vi "BRig_RT__Case_Exp__recordAnalogInput__PortC__dataQ.vi"(0 "input_dataAnalog":u16[][](array[numeric]), 1 "input_index":i32, 2 "input_iOccurence":u16, 3 "resetOccurrence":bool, 4 "input_dataCurrent":u16[](array[numeric]), 5 "input_stateList_NoInterrupt":u16[](array[numeric]), 6 "input_iState_start":T1, 7 "input_dataQ_hdl":refnum<queue>, 8 "input_iState_end":T1, 9 "input_dataQ_error":errorcluster, 10 "input_AI1":i16, 12 "input_AI0":i16) -> (11 "output_dataQ_error":errorcluster, 13 "output_dataQ_hdl":refnum<queue>, 14 "output_dataAnalog":u16[][](array[numeric]), 15 "output_index":i32, 16 "output_iOccurrence":u16)   [LabVIEW 2014]
uses:
  myRIO_BRig_RT__Case_Exp_stateList.ctl
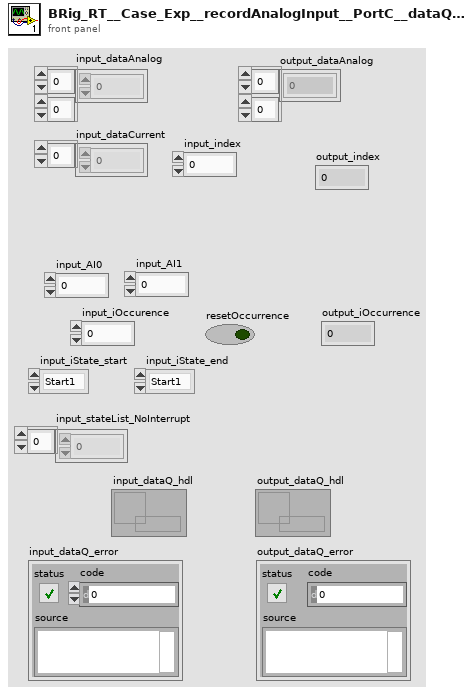
[diagram p1: front panel]
types:
  T1 = typedef "myRIO_BRig_RT__Case_Exp_stateList.ctl" = enum16{"Start1", "Start2", "Start3", "saveSettings1", "saveSettings2", "saveSettings3", "saveSettings4", "saveSettings_LC_ENL_l1", "saveSettings_LC_ENL_l2", "saveSettings_LC_Cue_l1", "saveSettings_LC_Cue_l2", "saveSettings6_LC_l1_Other", "SaveSettings6_LC_l2_Other", "setSettings_Audio", "setSettings_Laser", "initBlock_pre", "initBlock", "initBlock2", "initBlock_post", "initTrial_pre", "initTrial", "initTrial2", "initTrial3", "initTrial4", "initTrial_LC_ENL1", "initTrial_LC_Cue1", "initTrial_LC_Cue1_2", "initTrial_LC_Sel", "initTrial_post", "ENL1_pre", "ENL1", "ENL1_post", "ENL1Penalty_pre", "ENL1Penalty", "ENL2_pre", "ENL2", "ENL2Penalty_pre", "ENL2Penalty", "Cue1_pre", "Cue1", "Cue1_post", "Cue1Penalty_pre", "Cue1Penalty", "Cue2_pre", "Cue2", "Cue2Penalty_pre", "Cue2Penalty", "Selection_pre", "Selection", "Select_post", "SelectReward_pre", "SelectReward", "SelectRewardPost_pre", "SelectRewardPost", "SelectWrong_pre", "SelectWrong", "SelectWrong_post", "SelectTimeout_pre", "SelectTimeout", "SelectTimeout_post", "endTrial_pre", "endTrial1", "endTrial2", "endTrial3", "endTrial_post", "endBlock_pre", "endBlock", "endBlock_post", "endExp", "commConnect", "commUpload_pre", "commUpload_dataBlock", "commUpload_dataCurrent", "commUpload_dataExp", "commUpload_dataLC", "commUpload_dataTrial", "commUpload_post", "saveData_pre", "saveData_dataBlock", "saveData_dataCurrent", "saveData_dataExp", "saveData_dataLC", "saveData_dataTrial", "saveData_post", "empty_endBlock1", "empty_endBlock2", "empty_endTrial1", "empty_endTrial2", "empty_endTrial3", "empty_endTrial4", "empty_endTrial5", "dummyState", "dummyState_endBlock", "FreeReward_pre", "FreeReward", "FreeRewardPost_pre", "FreeRewardPost"}
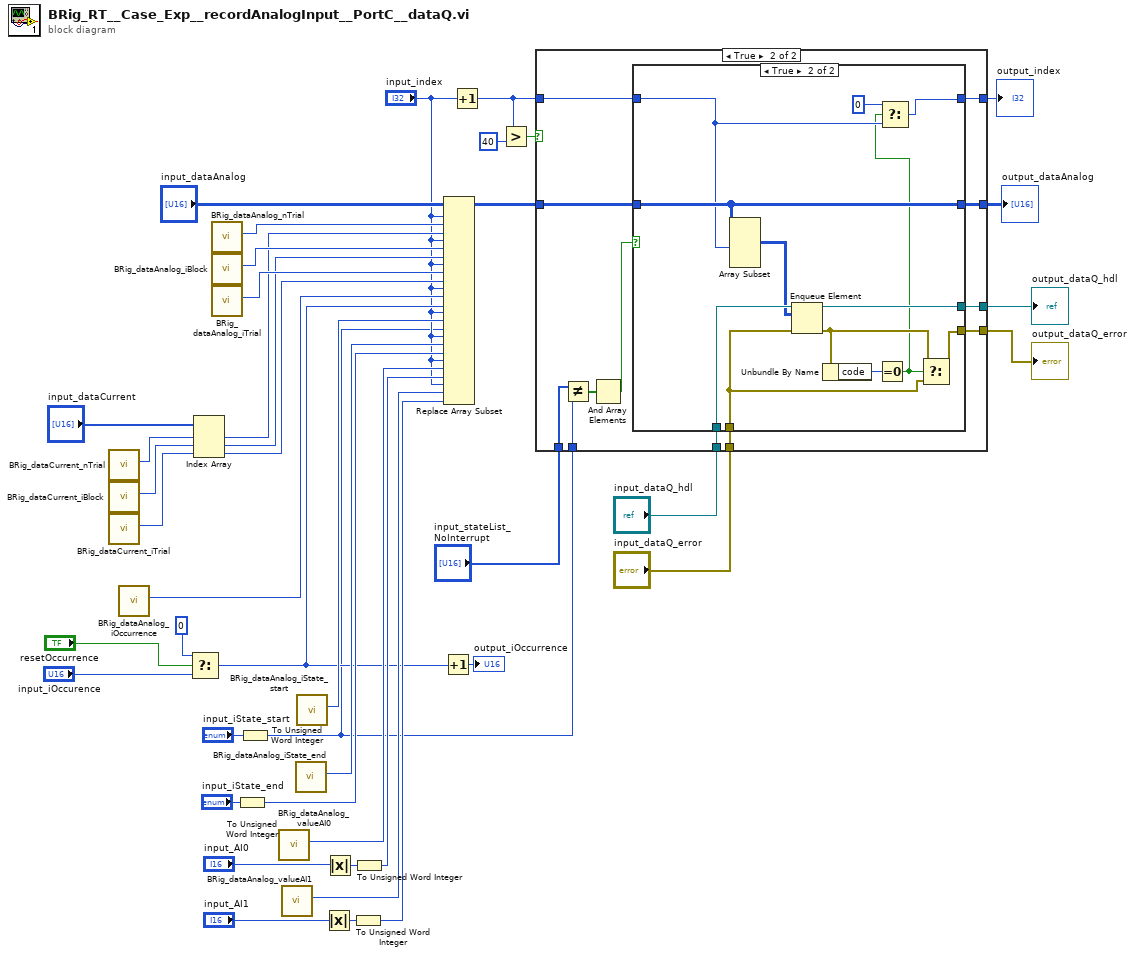
[diagram p0: block diagram]
diagram:
  n1 = call "BRig_dataCurrent_nTrial.vi"() -> ("output_nTrial"=w39:i32)  [unwired: 11 in]
  n2 = call "BRig_dataCurrent_iBlock.vi"() -> ("output_iBlock"=w38:i32)  [unwired: 11 in]
  n3 = call "BRig_dataCurrent_iTrial.vi"() -> ("output_iTrial"=w37:i32)  [unwired: 11 in]
  n4 = call "BRig_dataAnalog_iOccurrence.vi"() -> ("output_iOccurrence"=w30:i32)  [unwired: 11 in]
  n5 = Select(t=u16 0, s="resetOccurrence", f="input_iOccurence") -> (s? t:f=w21:u16)
  n6 = Index Array(array="input_dataCurrent", index #1=w39, index #2=w38, index #3=w37) -> (element #1=w15:u16, element #2=w16:u16, element #3=w14:u16)
  n7 = call "BRig_dataAnalog_nTrial.vi"() -> ("output_nTrial"=w36:i32)  [unwired: 11 in]
  n8 = call "BRig_dataAnalog_iBlock.vi"() -> ("output_iBlock"=w35:i32)  [unwired: 11 in]
  n9 = call "BRig_dataAnalog_iTrial.vi"() -> ("output_iTrial"=w34:i32)  [unwired: 11 in]
  n10 = To Unsigned Word Integer(number="input_iState_end") -> (unsigned 16bit integer=w29:u16)
  n11 = To Unsigned Word Integer(number="input_iState_start") -> (unsigned 16bit integer=w6:u16)
  n12 = call "BRig_dataAnalog_valueAI0.vi"() -> ("output_valueAI0"=w28:i32)  [unwired: 11 in]
  n13 = call "BRig_dataAnalog_valueAI1.vi"() -> ("output_valueAI1"=w27:i32)  [unwired: 11 in]
  n14 = call "BRig_dataAnalog_iState_end.vi"() -> ("output_iState_end"=w31:i32)  [unwired: 11 in]
  n15 = call "BRig_dataAnalog_iState_start.vi"() -> ("output_iState_start"=w32:i32)  [unwired: 11 in]
  n16 = Absolute Value(x="input_AI1") -> (abs(x)=w41:i16)
  n17 = Absolute Value(x="input_AI0") -> (abs(x)=w42:i16)
  n18 = To Unsigned Word Integer(number=w41) -> (unsigned 16bit integer=w25:u16)
  n19 = To Unsigned Word Integer(number=w42) -> (unsigned 16bit integer=w26:u16)
  n20 = Increment(x=w21) -> (x+1=→"output_iOccurrence":u16)
  n21 = Replace Array Subset(array="input_dataAnalog", new element #1=w15, index (row) #1="input_index", index (col) #1=w36, new element #2=w16, index (row) #2="input_index", index (col) #2=w35, new element #3=w14, index (row) #3="input_index", index (col) #3=w34, new element #4=w21, index (row) #4="input_index", index (col) #4=w30, new element #5=w6, index (row) #5="input_index", index (col) #5=w32, new element #6=w29, index (row) #6="input_index", index (col) #6=w31, new element #7=w26, index (row) #7="input_index", index (col) #7=w28, new element #8=w25, index (row) #8="input_index", index (col) #8=w27) -> (w10:u16[][])
  n22 = Increment(x="input_index") -> (x+1=w9:i32)
  n23 = Greater?(x=w9, y=40) -> (0:w11:bool)
  n24 = case shown="True" w11 {
    tunnel: w10 -> [w47 w58]
    tunnel: [w47 w58] -> w8
    tunnel: w9 -> [w46 w57]
    tunnel: [w46 w56] -> w7
    tunnel: w6 -> [_ w54]
    tunnel: "input_stateList_NoInterrupt" -> [_ w55]
    tunnel: "input_dataQ_hdl" -> [w45 w51]
    tunnel: "input_dataQ_error" -> [w44 w50]
    tunnel: [w45 w49] -> w2
    tunnel: [w44 w48] -> w1
    frame False {
    }
    frame True {
      n25 = Not Equal?(x=w55, y=w54) -> (x != y?=w53:bool[])
      n26 = And Array Elements(Boolean array=w53) -> (logical AND=w52:bool)
      n27 = case shown="True" w52 {
        tunnel: w58 -> [w61 w71]
        tunnel: w57 -> [w62 w74]
        tunnel: [w62 w72] -> w56
        tunnel: [w61 w71] -> _
        tunnel: w51 -> [w59 w70]
        tunnel: w50 -> [w60 w64]
        tunnel: [w59 w68] -> w49
        tunnel: [w60 w65] -> w48
        frame False {
        }
        frame True {
          n28 = Array Subset(array=w71, length (row)=w74) -> (w69:u16[][])  [unwired: 3 in]
          n29 = Enqueue Element(queue=w70, element=w69, error in (no error)=w64) -> (queue out=w68:refnum<queue>, error out=w66:errorcluster)  [unwired: 1 in, 1 out]
          n30 = Unbundle By Name(w66) -> ("code"=w67:i32)
          n31 = Equal To 0?(x=w67) -> (x = 0?=w63:bool)
          n32 = Select(t=0, s=w63, f=w74) -> (s? t:f=w72:i32)
          n33 = Select(t=w66, s=w63, f=w64) -> (s? t:f=w65:errorcluster)
        }
      }
    }
  }
  "output_dataAnalog" <- w8
  "output_index" <- w7
  "output_dataQ_hdl" <- w2
  "output_dataQ_error" <- w1
